vi "event_structure_playground.vi"() -> ()   [LabVIEW 2010]
panel:
  in  "Number of Repeats":i32=1
  in  "stop":bool
  in  "DataFile":path
  in  "Start Run":bool
  out "Randnum":dbl
  out "x > y?":bool
  in  "Stop this VI":bool
  in  "?":bool
  # "Try to close this front panel \nwhile the VI is running."
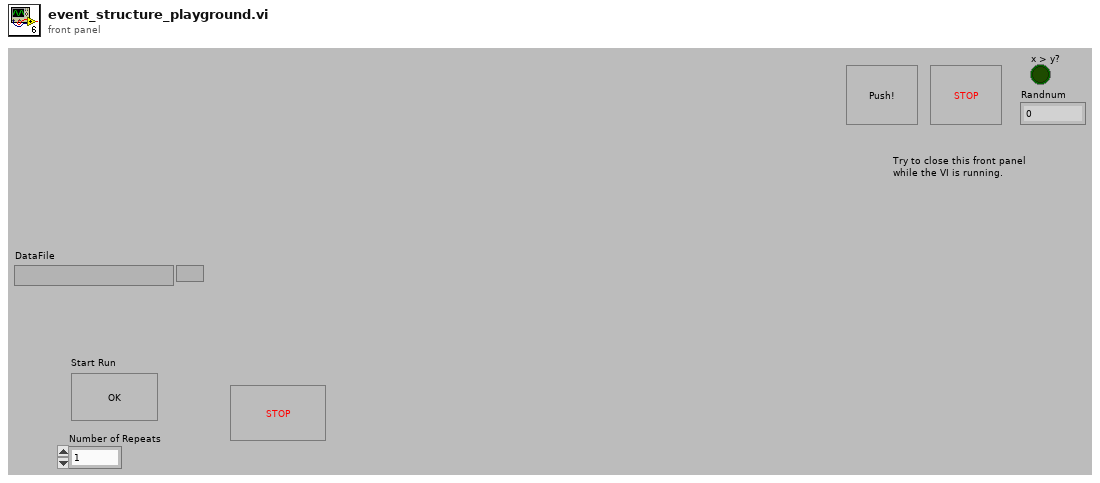
[diagram p1: front panel]
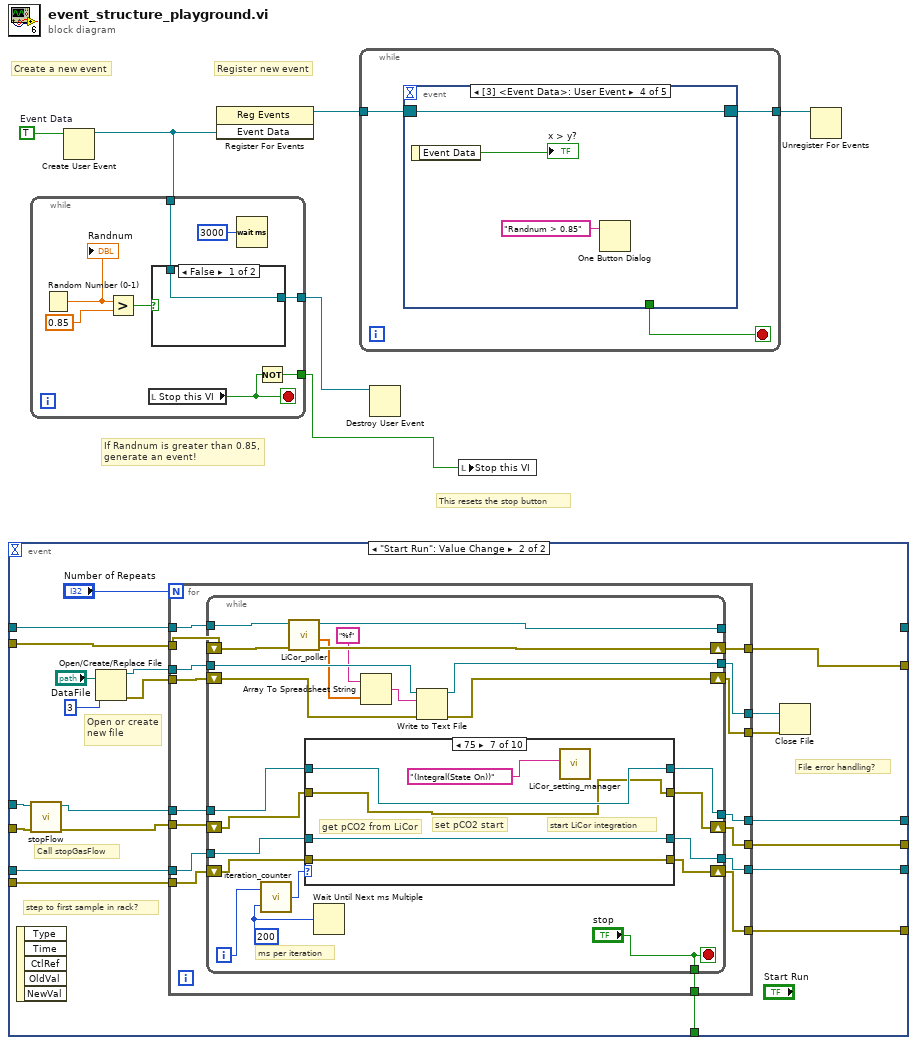
[diagram p0: block diagram]
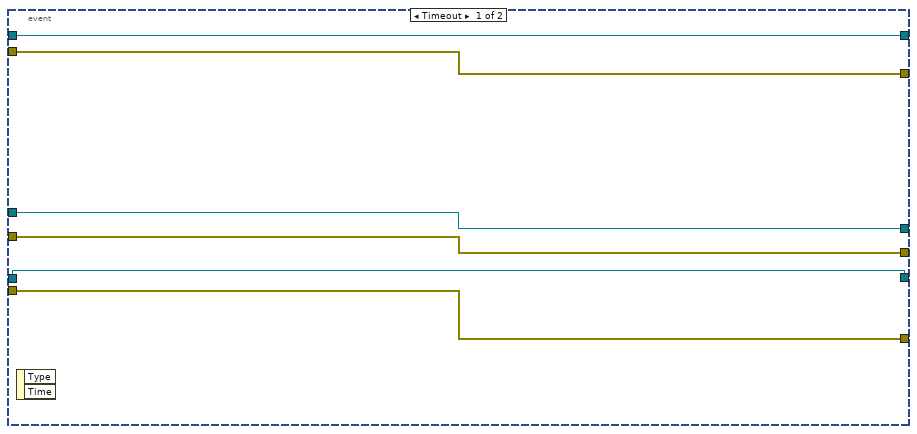
[diagram p2: hidden frame]
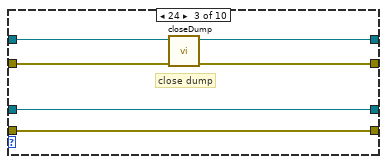
[diagram p5: hidden frame]
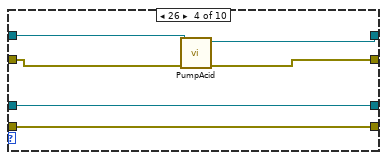
[diagram p6: hidden frame]
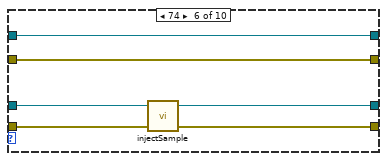
[diagram p8: hidden frame]
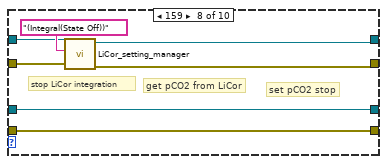
[diagram p9: hidden frame]
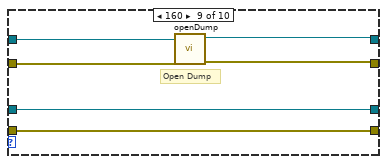
[diagram p10: hidden frame]
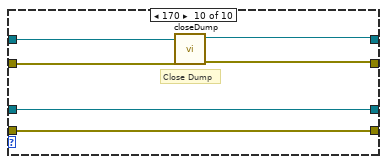
[diagram p11: hidden frame]
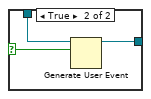
[diagram p12: hidden frame]
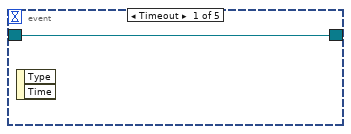
[diagram p13: hidden frame]
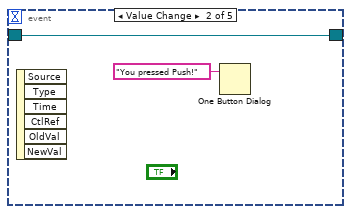
[diagram p14: hidden frame]
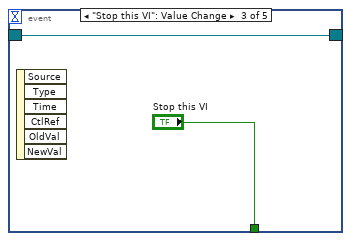
[diagram p15: hidden frame]
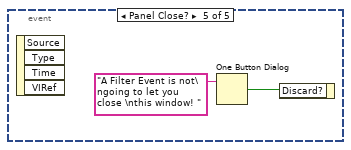
[diagram p16: hidden frame]
diagram:
  w6 = TRUE  # Event Data
  # "Register new event"
  # "Create a new event"
  # "This resets the stop button"
  # "If Randnum is greater than 0.85,\ngenerate an event!"
  n1 = event shown="[1] \"Start Run\": Value Change" {
    selector: _ -> [_ _]
    dyn-events: _ -> [_ _]
    timeout: _ -> [_ _]
    tunnel: _ -> [w11 w32]
    tunnel: _ -> [w12 w31]
    tunnel: _ -> [w10 w25]
    tunnel: _ -> [w9 w24]
    tunnel: _ -> [w8 w19]
    tunnel: _ -> [w7 w18]
    tunnel: [_ w20] -> _
    tunnel: [w12 w17] -> _
    tunnel: [w11 _] -> _
    tunnel: [w10 w16] -> _
    tunnel: [w9 w15] -> _
    tunnel: [w8 w14] -> _
    tunnel: [w7 w13] -> _
    event Timeout {
      n2 = event-data() -> ()  [unwired: 1 in, 2 out]
    }
    event "Start Run": Value Change {
      # "File error handling?"
      # "Call stopGasFlow"
      # "step to first sample in rack?"
      # "Open or create new file"
      n3 = event-data() -> ()  [unwired: 1 in, 5 out]
      n4 = call "stopFlow.vi"("error in"=w24, "VISA resource name"=w25) -> ("error out"=w26:errorcluster, "VISA resource out"=w27:refnum<visa-resource-name>)  [unwired: 8 in]
      n5 = Open/Create/Replace File(file path (use dialog)="DataFile", operation (0:open)=3) -> (refnum out=w28:refnum<file>, error out=w23:errorcluster)  [unwired: 4 in, 1 out]
      n6 = for {
        N: "Number of Repeats" -> [_]
        tunnel: w32 -> [w49]
        tunnel: w31 -> [w48]
        tunnel: w28 -> [w47]
        tunnel: w27 -> [w45]
        tunnel: w26 -> [w46]
        tunnel: w23 -> [w44]
        tunnel: [w43] -> w22
        tunnel: [w42] -> w21
        tunnel: [w41] -> w20
        tunnel: w19 -> [w40]
        tunnel: w18 -> [w39]
        tunnel: [w38] -> w17
        tunnel: [w37] -> w16
        tunnel: [w36] -> w15
        tunnel: [w35] -> w14
        tunnel: [w34] -> w13
        n7 = while {
          tunnel: [w72] -> _
          tunnel: w49 -> [w71]
          shift-right: [w69] -> w38
          shift-left: w48 -> [w70]
          tunnel: w47 -> [w68]
          tunnel: w45 -> [w61]
          tunnel: [w64] -> w43
          shift-right: [w63] -> w42
          shift-left: w44 -> [w67]
          tunnel: ["stop"] -> w41
          tunnel: w40 -> [w59]
          shift-right: [w57] -> w34
          shift-left: w39 -> [w58]
          tunnel: [w56] -> w35
          tunnel: [w55] -> w37
          shift-right: [w54] -> w36
          shift-left: w46 -> [w60]
          i -> [w52]
          stop <- "stop" stop-if-true
          w51 = 200 ("ms between samples")
          # "ms per iteration"
          n8 = call "iteration_counter.vi"("ms per iteration"=w51, "index"=w52) -> ("seconds"=w53:i32)
          n9 = call "LiCor_poller.vi"("error in"=w70, "VISA session in"=w71) -> ("error out"=w69:errorcluster, "data array"=w66:dbl[], "VISA session out"=w72:refnum<visa-resource-name>)  [unwired: 5 in, 2 out]
          n10 = case shown="75" w53 {
            tunnel: w61 -> [w74 w78 w84 w90 w96 w102 w105 w111 w118 w124]
            tunnel: w60 -> [w73 w77 w82 w89 w95 w101 w104 w108 w117 w123]
            tunnel: w59 -> [w76 w80 w85 w92 w94 w100 w107 w114 w120 w126]
            tunnel: w58 -> [w75 w79 w86 w91 w93 w99 w106 w113 w119 w125]
            tunnel: [w75 w79 w86 w91 w93 w97 w106 w113 w119 w125] -> w57
            tunnel: [w76 w80 w85 w92 w94 w98 w107 w114 w120 w126] -> w56
            tunnel: [w74 w78 w83 w88 w96 w102 w105 w110 w115 w121] -> w55
            tunnel: [w73 w77 w81 w87 w95 w101 w104 w109 w116 w122] -> w54
            frame 0, Default {
            }
            frame 1 {
              # "Run Rinse_GetSample"
            }
            frame 24 {
              # "close dump"
              n11 = call "closeDump.vi"("error in"=w82, "VISA resource name"=w84) -> ("error out"=w81:errorcluster, "VISA resource out"=w83:refnum<visa-resource-name>)  [unwired: 8 in]
            }
            frame 26 {
              n12 = call "PumpAcid.vi"("error in"=w89, "VISA resource name"=w90) -> ("error out"=w87:errorcluster, "VISA resource out"=w88:refnum<visa-resource-name>)  [unwired: 8 in]
            }
            frame 60 {
              # "normal flow"
            }
            frame 74 {
              n13 = call "injectSample.vi"("error in"=w99, "VISA resource in"=w100) -> ("error out"=w97:errorcluster, "VISA resource out"=w98:refnum<visa-resource-name>)  [unwired: 2 in]
            }
            frame 75 {
              # "start LiCor integration"
              # "set pCO2 start"
              # "get pCO2 from LiCor"
              n14 = call "LiCor_setting_manager.vi"("string to write"="(Integral(State On))") -> ()  [unwired: 9 in, 2 out]
            }
            frame 159 {
              # "set pCO2 stop"
              # "get pCO2 from LiCor"
              # "stop LiCor integration"
              n15 = call "LiCor_setting_manager.vi"("error in"=w108, "string to write"="(Integral(State Off))", "VISA session in"=w111) -> ("error out"=w109:errorcluster, "VISA session out"=w110:refnum<visa-resource-name>)  [unwired: 7 in]
            }
            frame 160 {
              # "Open Dump"
              n16 = call "openDump.vi"("error in"=w117, "VISA resource name"=w118) -> ("error out"=w116:errorcluster, "VISA resource out"=w115:refnum<visa-resource-name>)  [unwired: 8 in]
            }
            frame 170 {
              # "Close Dump"
              n17 = call "closeDump.vi"("error in"=w123, "VISA resource name"=w124) -> ("error out"=w122:errorcluster, "VISA resource out"=w121:refnum<visa-resource-name>)  [unwired: 8 in]
            }
          }
          n18 = Wait Until Next ms Multiple(millisecond multiple=w51) -> ()  [unwired: 1 out]
          n19 = Array To Spreadsheet String(array=w66, 3:"%f") -> (spreadsheet string=w65:string)  [unwired: 1 in]
          n20 = Write to Text File(file (use dialog)=w68, text=w65, error in=w67) -> (refnum out=w64:refnum<file>, error out=w63:errorcluster)  [unwired: 1 in, 1 out]
        }
      }
      n21 = Close File(refnum=w22, error in=w21) -> ()  [unwired: 2 out]
    }
  }
  n22 = Create User Event(user event datatype=w6) -> (user event=w3:refnum<user-event>)  [unwired: 1 in, 1 out]
  n23 = while {
    tunnel: w3 -> [w128]
    tunnel: [w130] -> w2
    tunnel: [w127] -> w1
    stop <- w131 stop-if-true
    n24 = Random Number (0-1)() -> (number: 0 to 1=w134:dbl)
    "Randnum" <- w134
    n25 = Greater?(x=w134, y=0.85) -> (0:w129:bool)
    n26 = local read "Stop this VI"() -> (w131:bool)
    n27 = case shown="False" w129 {
      selector: w129 -> [_ w137]
      tunnel: w128 -> [w135 w138]
      tunnel: [w135 w136] -> w127
      frame False {
      }
      frame True {
        n28 = Generate User Event(user event=w138, event data cluster=w137) -> (user event out=w136:refnum<user-event>)  [unwired: 1 in, 1 out]
      }
    }
    n29 = Wait (ms)(milliseconds to wait=u32 3000) -> ()  [unwired: 1 out]
    n30 = Not(x=w131) -> (.not. x?=w130:bool)
  }
  n31 = register-events(w3) -> (reference out=w5:refnum<event-registration>)  [unwired: 2 in, 1 out]
  n32 = while {
    tunnel: w5 -> [w140]
    tunnel: [w139] -> w4
    stop <- w141 stop-if-true
    n33 = event shown="[3] <Event Data>: User Event" {
      selector: w140 -> [w142 w143 w145 w149 _]
      dyn-events: [w142 w143 w145 w149 _] -> w139
      timeout: _ -> [_ _ _ _ _]
      tunnel: [_ _ "Stop this VI" _ _] -> w141
      event Timeout {
        n34 = event-data() -> ()  [unwired: 1 in, 2 out]
      }
      event Value Change {
        n35 = event-data() -> ()  [unwired: 1 in, 6 out]
        n36 = One Button Dialog(message="You pressed Push!") -> ()  [unwired: 1 in, 1 out]
      }
      event "Stop this VI": Value Change {
        n37 = event-data() -> ()  [unwired: 1 in, 6 out]
      }
      event User Event {
        n38 = event-data() -> ("Event Data"=→"x > y?":bool)  [unwired: 1 in]
        n39 = One Button Dialog(message="Randnum > 0.85") -> ()  [unwired: 1 in, 1 out]
      }
      event Panel Close? {
        n40 = event-data() -> ()  [unwired: 1 in, 4 out]
        n41 = One Button Dialog(message="A Filter Event is not\ngoing to let you close \nthis window! ") -> (true=w150:bool)  [unwired: 1 in]
        n42 = event-data("Discard?"=w150) -> ()  [unwired: 1 in, 1 out]
      }
    }
  }
  n43 = Destroy User Event(user event=w1) -> ()  [unwired: 1 in, 1 out]
  n44 = local write "Stop this VI"(w2) -> ()
  n45 = Unregister For Events(event registration refnum=w4) -> ()  [unwired: 1 in, 1 out]
